vi "Data_Table.vi"(9 "AllControls In":T1, 11 "Data in":T2) -> (3 "Data out":string[][](array[string]))   [LabVIEW 2017]
uses:
  Ctrls/CSV_Data.ctl
  Ctrls/AllControls.ctl
panel:
  out "大小 2":i32[](array[numeric])
  out "大小":i32
  out "数组":string[](array[string])
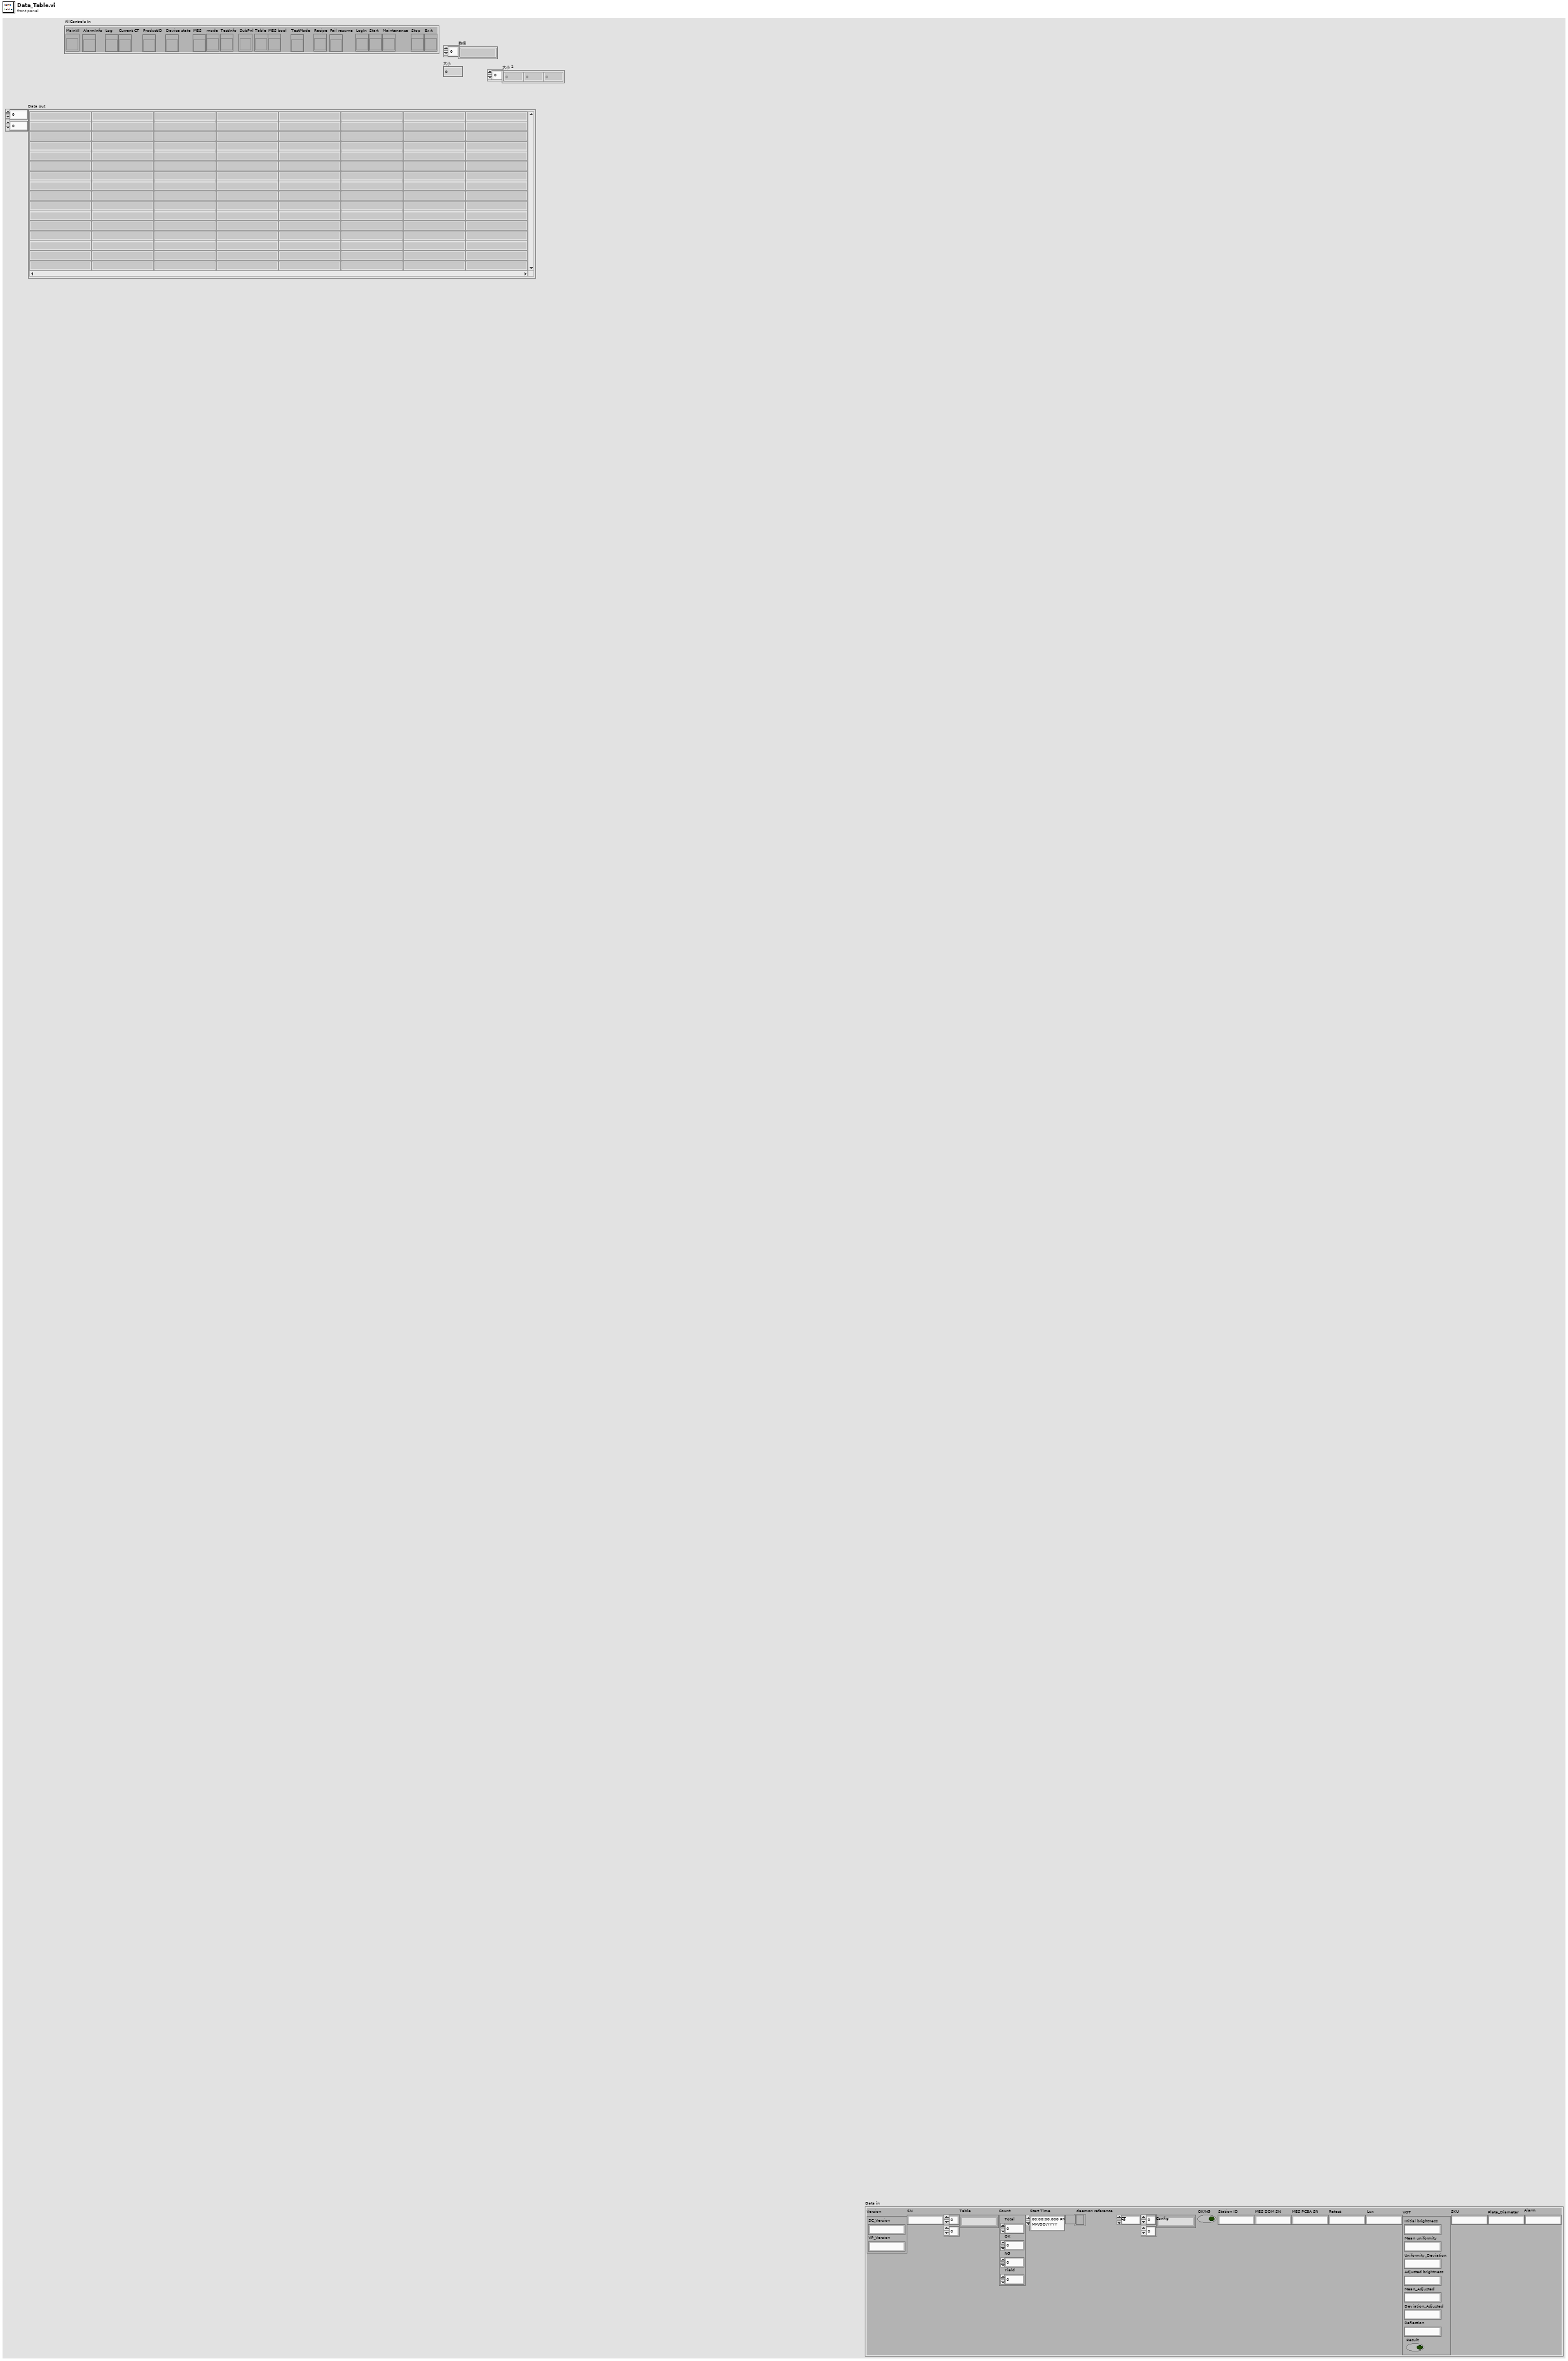
[diagram p1: front panel]
types:
  T1 = typedef "AllControls.ctl" = cluster{"MainVI":refnum<vi>, "AlarmInfo":refnum<vi>, "Log":refnum<vi>, "Current CT":refnum<vi>, "ProductID":refnum<vi>, "Device state":refnum<vi>, "MES":refnum<vi>, "mode":refnum<vi>, "TestInfo":refnum<vi>, "SubPnl":refnum<vi>, "Table":refnum<vi>, "MES bool":refnum<vi>, "TestMode":refnum<vi>, "Recipe":refnum<vi>, "Fail resume":refnum<vi>, "LogIn":refnum<vi>, "Start":refnum<vi>, "Maintenance":refnum<vi>, "Stop":refnum<vi>, "Exit":refnum<vi>}
  T2 = typedef "CSV_Data.ctl" = cluster{"Version":cluster{"SC_Version":string, "VP_Version":string}, "SN":string, "Table":string[][], "Count":cluster{"Total":i32, "OK":i32, "NG":i32, "Yield":dbl}, "Start Time":timestamp, "daemon reference":refnum<k5>, "CT":dbl, "Config":string[][], "OK/NG":bool, "Station ID":string, "MES DDM SN":string, "MES PCBA SN":string, "Retest":string, "Lux":string, "VOT":cluster{"Initial brightness":string, "Mean uniformity":string, "Uniformity_Deviation":string, "Adjusted brightness":string, "Mean_Adjusted":string, "Deviation_Adjusted":string, "Reflection":string, "Result":bool}, "SKU":string, "Plate_Diameter":string, "Alarm":string}
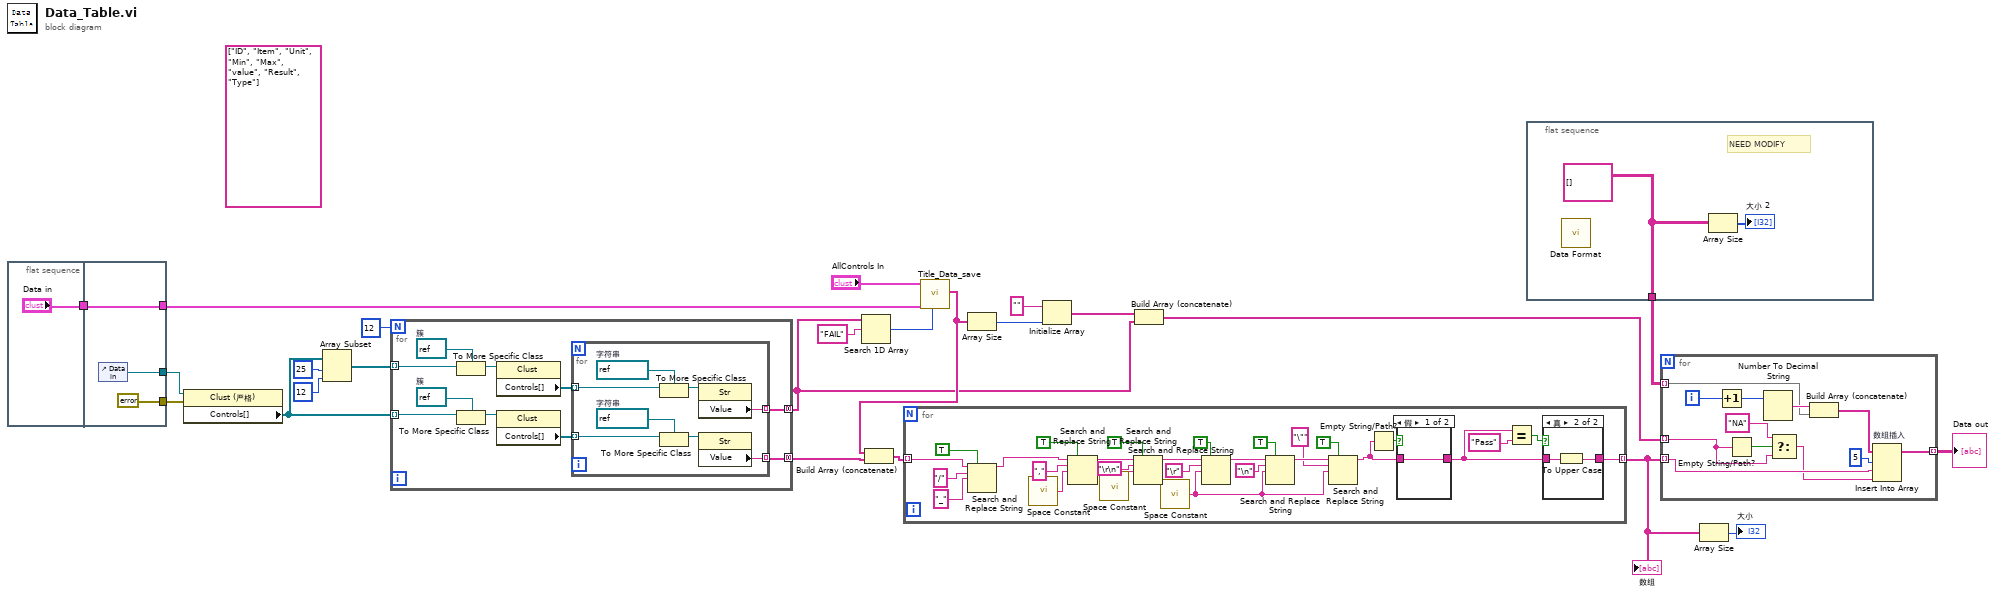
[diagram p0: block diagram]
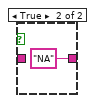
[diagram p3: hidden frame]
diagram:
  (unwired) string[] ["ID", "Item", "Unit", "Min", "Max", "value", "Result", "Type"] ("列首字符串[]")
  n1 = flat-sequence {
    tunnel: ["Data in"] -> w23
    tunnel: [w28] -> w12
    tunnel: w23 -> [w28]
    tunnel: [errorcluster {"status"=FALSE, "code"=0, "source"=""} ("错误输入（无错误）")] -> w17
    tunnel: [w26] -> w16
    frame #0 {
    }
    frame #1 {
      n2 = control-ref of="Data in"() -> (w26:refnum<vi>)
    }
  }
  n3 = property class="Clust (严格)"(reference=w16, error in=w17) -> ("Controls[]"=w21:refnum<vi>[])  [unwired: 2 out]
  n4 = Array Subset(array=w21, index=25 ("索引"), length=12 ("长度")) -> (w18:refnum<vi>[])
  n5 = for {
    N: 12 -> [_]
    tunnel: w21 -> [w38] mode=indexing
    tunnel: [w34] -> w9 mode=concatenating
    tunnel: w18 -> [w31] mode=indexing
    tunnel: [w29] -> w3 mode=concatenating
    w32 = refnum<vi> refnum  # 簇
    w37 = refnum<vi> refnum  # 簇
    n6 = To More Specific Class(target class=w32, reference=w31) -> (specific class reference=w33:refnum<vi>)  [unwired: 1 in, 1 out]
    n7 = To More Specific Class(target class=w37, reference=w38) -> (specific class reference=w36:refnum<vi>)  [unwired: 1 in, 1 out]
    n8 = property class="Clust"(reference=w33) -> ("Controls[]"=w30:refnum<vi>[])  [unwired: 1 in, 2 out]
    n9 = property class="Clust"(reference=w36) -> ("Controls[]"=w35:refnum<vi>[])  [unwired: 1 in, 2 out]
    n10 = for {
      tunnel: w35 -> [w45] mode=indexing
      tunnel: [w43] -> w34 mode=indexing
      tunnel: w30 -> [w40] mode=indexing
      tunnel: [w39] -> w29 mode=indexing
      w41 = refnum<vi> refnum  # 字符串
      w46 = refnum<vi> refnum  # 字符串
      n11 = To More Specific Class(target class=w41, reference=w40) -> (specific class reference=w42:refnum<vi>)  [unwired: 1 in, 1 out]
      n12 = To More Specific Class(target class=w46, reference=w45) -> (specific class reference=w44:refnum<vi>)  [unwired: 1 in, 1 out]
      n13 = property class="Str"(reference=w42) -> ("Value"=w39:string)  [unwired: 1 in, 2 out]
      n14 = property class="Str"(reference=w44) -> ("Value"=w43:string)  [unwired: 1 in, 2 out]
    }
  }
  n15 = Search 1D Array(1D array=w3, element="FAIL") -> (index of element=w11:i32)  [unwired: 1 in]
  n16 = call "Title_Data_save.vi"("ErrorIndex"=w11, "Data in"=w12, "AllControls In"="AllControls In") -> ("数组"=w7:string[])  [unwired: 8 in]
  n17 = Build Array (concatenate)(w7, w9) -> (w8:string[])
  n18 = for {
    tunnel: w8 -> [w48] mode=indexing
    tunnel: [w59] -> w15 mode=indexing
    n19 = Search and Replace String(replace all?=TRUE ("replace all? (F)"), input string=w48, search string="/", replace string="_") -> (result string=w47:string)  [unwired: 4 in, 3 out]
    n20 = call <vilib>:"Space Constant.vi"() -> ("String"=w72:string)
    n21 = Search and Replace String(replace all?=TRUE ("replace all? (F)"), input string=w47, search string=",", replace string=w72) -> (result string=w65:string)  [unwired: 4 in, 3 out]
    n22 = call <vilib>:"Space Constant.vi"() -> ("String"=w71:string)
    n23 = Search and Replace String(replace all?=TRUE ("replace all? (F)"), input string=w65, search string="\r\n", replace string=w71) -> (result string=w70:string)  [unwired: 4 in, 3 out]
    n24 = call <vilib>:"Space Constant.vi"() -> ("String"=w53:string)
    n25 = Search and Replace String(replace all?=TRUE ("replace all? (F)"), input string=w70, search string="\r", replace string=w53) -> (result string=w64:string)  [unwired: 4 in, 3 out]
    n26 = Search and Replace String(replace all?=TRUE ("替换全部？(F)"), input string=w64, search string="\n", replace string=w53) -> (result string=w55:string)  [unwired: 4 in, 3 out]
    n27 = Search and Replace String(replace all?=TRUE ("替换全部？(F)"), input string=w55, search string="\"", replace string=w53) -> (result string=w54:string)  [unwired: 4 in, 3 out]
    n28 = Empty String/Path?(string/path=w54) -> (empty?=w61:bool)
    n29 = case shown="假" w61 {
      tunnel: [w78 "NA" ("x")] -> w60
      tunnel: w54 -> [w78 _]
      frame False {
      }
      frame True {
      }
    }
    n30 = Equal?(x=w60, y="Pass") -> (x = y?=w57:bool)
    n31 = case shown="真" w57 {
      tunnel: [w75 w77] -> w59
      tunnel: w60 -> [w75 w76]
      frame False {
      }
      frame True {
        n32 = To Upper Case(1:w76) -> (0:w77:string)
      }
    }
  }
  "数组" <- w15
  n33 = Array Size(array=w7) -> (size(s)=w6:i32)
  n34 = Initialize Array("", w6) -> (w4:string[])
  n35 = Build Array (concatenate)(w4, w3) -> (w2:string[])
  n36 = flat-sequence {
    tunnel: [w80] -> w1
    frame #0 {
      w80 = string[][] [] ("数组")
      # "NEED MODIFY"
      n37 = call "Data Format.vi"() -> ()  [unwired: 10 in, 2 out]
      n38 = Array Size(array=w80) -> (size(s)=→"大小 2":i32[])
    }
  }
  n39 = for {
    tunnel: [w88] -> w24 mode=indexing
    tunnel: w1 -> [w91] mode=indexing
    tunnel: w15 -> [w86] mode=indexing
    tunnel: w2 -> [w84] mode=indexing
    i -> [w87]
    n40 = Increment(x=w87) -> (x+1=w93:i32)
    n41 = Empty String/Path?(string/path=w84) -> (empty?=w85:bool)
    n42 = Number To Decimal String(number=w93) -> (decimal integer string=w92:string)  [unwired: 1 in]
    n43 = Select(t="NA", s=w85, f=w84) -> (s? t:f=w82:string)
    n44 = Build Array (concatenate)(w92, w91) -> (w90:string[])
    n45 = Insert Into Array "数组插入"(array=w90, index=5 ("索引"), new element #1=w86, new element #2=w82) -> (w88:string[])
  }
  "Data out" <- w24
  n46 = Array Size(array=w15) -> (size(s)=→"大小":i32)
